vi "SonarRefNum_Simulation_Global.vi"(0 "menu":enum16{"set", "get", "delete"}(ring)=enum."get", 1 "Ping DIO Channel":T1=enum."DIO 1", 7 "Echo DIO Channel":T1=enum."DIO 2", 9 "Devantech SRF05 Set":refnum<class "Devantech SRF05.lvclass">, 11 "error in (no error)":errorcluster) -> (10 "Devantech SRF05 Get":refnum<class "Devantech SRF05.lvclass">, 15 "error out":errorcluster)   [LabVIEW 2017]
doc: "Sets a reference into a registry, gets a reference from a registry, or deletes a reference from a registry. The reference is accessed by name, and can be given any unique name.\n\nThis software is licensed. Open the labview\\readme\\WPI Robotics Library Open Source License.txt file for more information."
uses:
  <vilib>/Rock Robotics/SystemInterfaces/DIO/FPGA_DIOChannel.ctl
  <instrlib>/Devantech SRF05/HAIOL/Devantech SRF05.lvclass
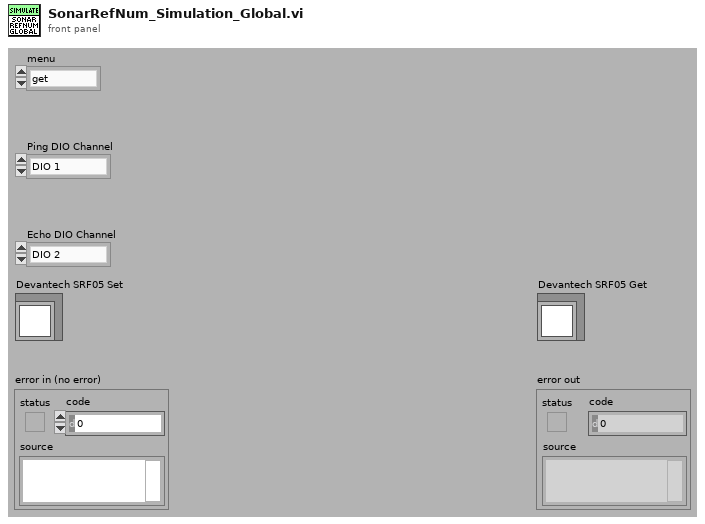
[diagram p1: front panel]
types:
  T1 = typedef "FPGA_DIOChannel.ctl" = enum8{"DIO 0", "DIO 1", "DIO 2", "DIO 3", "DIO 4", "DIO 5", "DIO 6", "DIO 7", "DIO 8", "DIO 9", "DIO MXP 0", "DIO MXP 1", "DIO MXP 2", "DIO MXP 3", "DIO MXP 4", "DIO MXP 5", "DIO MXP 6", "DIO MXP 7", "DIO MXP 8", "DIO MXP 9", "DIO MXP 10", "DIO MXP 11", "DIO MXP 12", "DIO MXP 13", "DIO MXP 14", "DIO MXP 15", "SPI Port CS1", "SPI Port CS2", "SPI Port CS3", "SPI Port MISO", "SPI Port MOSI", "Invalid"}
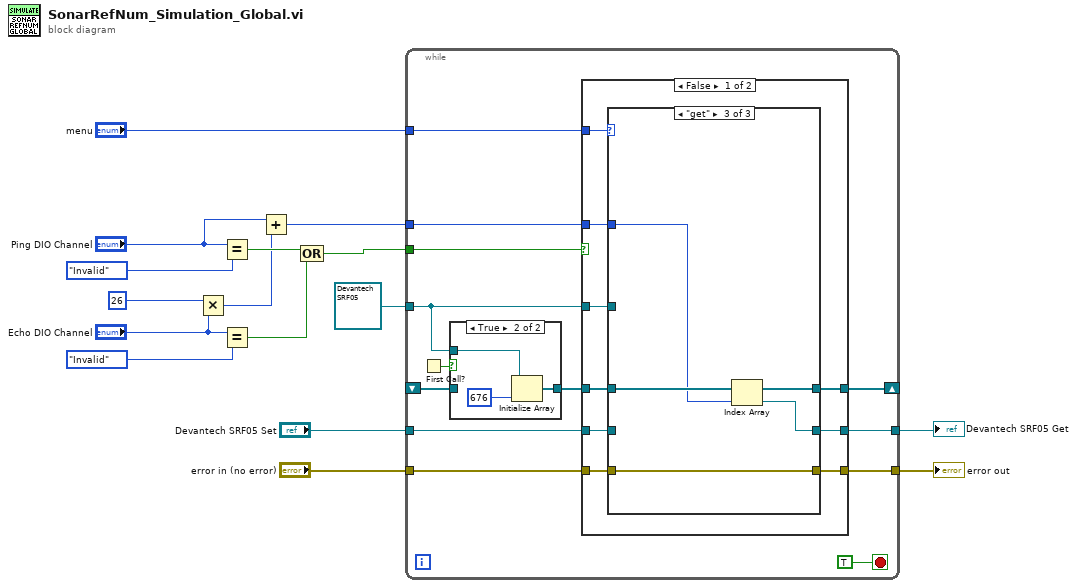
[diagram p0: block diagram]
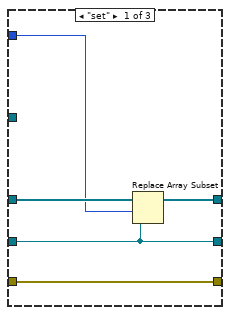
[diagram p2: hidden frame]
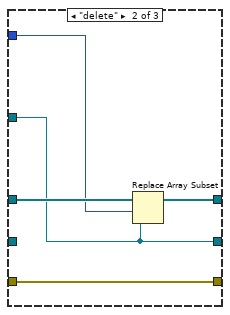
[diagram p3: hidden frame]
diagram:
  n1 = Multiply(x=u16 26 ("x*y"), y="Echo DIO Channel") -> (x*y=w5:u16)
  n2 = Equal?(x="Ping DIO Channel", y=FPGA_DIOChannel."Invalid" ("Echo DIO Channel")) -> (x = y?=w13:bool)
  n3 = Equal?(x="Echo DIO Channel", y=FPGA_DIOChannel."Invalid" ("Echo DIO Channel")) -> (x = y?=w7:bool)
  n4 = Add(x="Ping DIO Channel", y=w5) -> (x+y=w6:u16)
  n5 = Compound Arithmetic op=OR(w13, w7) -> (w8:bool)
  n6 = while {
    tunnel: "Devantech SRF05 Set" -> [w29]
    tunnel: "error in (no error)" -> [w25]
    shift-right: [w28] -> _
    shift-left: _ -> [w20]
    tunnel: [w27] -> w11
    tunnel: "menu" -> [w26]
    tunnel: [w24] -> w15
    tunnel: w6 -> [w19]
    tunnel: w8 -> [w18]
    tunnel: refnum<class "Devantech SRF05.lvclass"> refnum ("Devantech SRF05 out") -> [w17]
    stop <- TRUE stop-if-true
    n7 = First Call?() -> (First Call?: T/F=w22:bool)
    n8 = case shown="True" w22 {
      tunnel: [w56 w58] -> w21
      tunnel: w20 -> [w56 _]
      tunnel: w17 -> [_ w57]
      frame False {
      }
      frame True {
        n9 = Initialize Array(w57, 676 ("dimension size")) -> (w58:refnum<class "Devantech SRF05.lvclass">[])
      }
    }
    n10 = case shown="False" w18 {
      tunnel: w29 -> [w38 _]
      tunnel: [w37 w55] -> w28
      tunnel: [w36 w53] -> w27
      tunnel: w26 -> [w35 _]
      tunnel: w25 -> [w34 w54]
      tunnel: [w33 w54] -> w24
      tunnel: w21 -> [w32 w55]
      tunnel: w19 -> [w31 _]
      tunnel: w17 -> [w30 w53]
      frame False {
        n11 = case shown="\"get\"" w35 {
          tunnel: w38 -> [w41 _ _]
          tunnel: [w42 w47 w52] -> w37
          tunnel: w32 -> [w43 w48 w52]
          tunnel: [w41 w44 w51] -> w36
          tunnel: [w40 w46 w50] -> w33
          tunnel: w34 -> [w40 w46 w50]
          tunnel: w31 -> [w39 w45 w49]
          tunnel: w30 -> [_ w44 _]
          frame "set" {
            n12 = Replace Array Subset(array=w43, new element=w41, index=w39) -> (w42:refnum<class "Devantech SRF05.lvclass">[])
          }
          frame "delete" {
            n13 = Replace Array Subset(array=w48, new element=w44, index=w45) -> (w47:refnum<class "Devantech SRF05.lvclass">[])
          }
          frame "get" {
            n14 = Index Array(array=w52, index=w49) -> (element=w51:refnum<class "Devantech SRF05.lvclass">)
          }
        }
      }
      frame True {
        # "Do nothing if channel is Invalid."
      }
    }
  }
  "error out" <- w15
  "Devantech SRF05 Get" <- w11
